vi "Configure Power Supply Rejection Ratio Analysis (Frequency).vi"(6 "Maximum Frequency (7: 20000000 Hz)":i32(ring)=7 items=["10", "100", "1000", "10000", "100000", "1000000", "10000000", "20000000"], 7 "Single Frequency (2: 100 Hz)":i32(ring)=2 items=["1", "10", "100", "1000", "10000", "100000", "1000000", "10000000", "2000000"], 8 "error in (no error)":errorcluster, 9 "Minimum Frequency (2: 100 Hz)":i32(ring)=2 items=["1", "10", "100", "1000", "10000", "100000", "1000000", "10000000", "2000000"], 10 "Frequency Mode (0: Sweep)":i32(ring) items=["Sweep", "Single"], 11 "VISA resource name":refnum<visa-resource-name>) -> (0 "error out":errorcluster, 3 "VISA resource name out":refnum<visa-resource-name>)   [LabVIEW 2015, in "Agilent 2000 3000 X-Series.lvlib"]
doc: "Configures the frequency for Power Supply Rejection Ratio (PSRR) power analysis.\n\n<b>Note:</b>\n - This VI is applicable for 3000T, 3000G, 4000, 6000 X-Series."
uses:
  Agilent 2000 3000 X-Series.lvlib
panel:
  # "Single Mode"
  # "Sweep Mode"
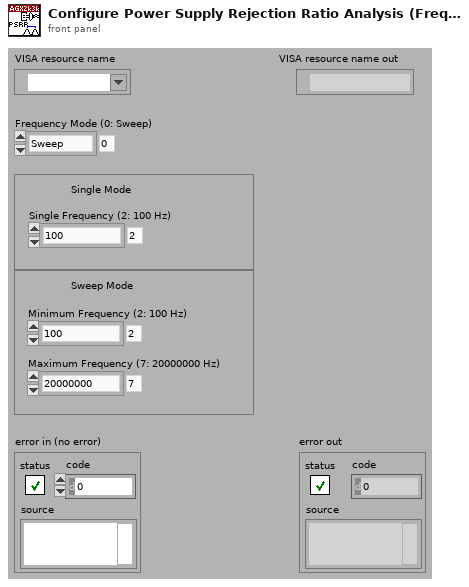
[diagram p1: front panel]
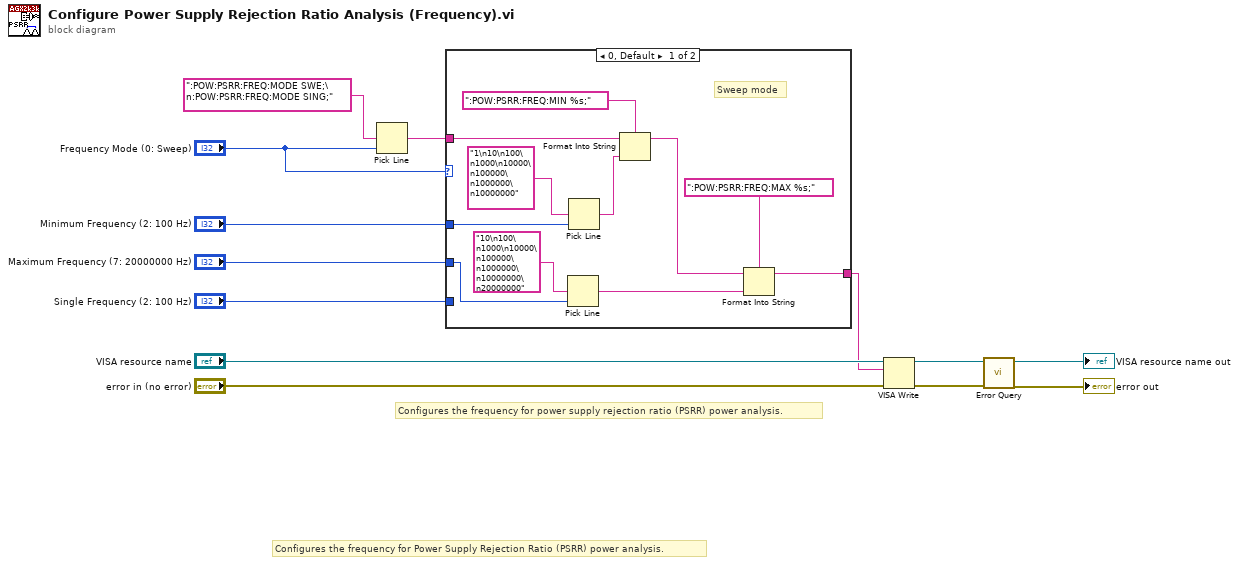
[diagram p0: block diagram]
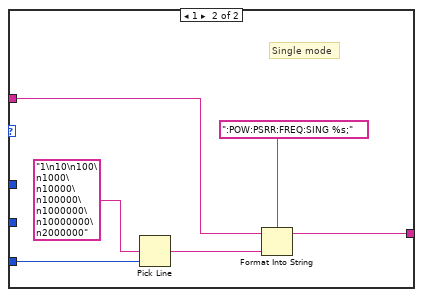
[diagram p2: hidden frame]
diagram:
  # "Configures the frequency for power supply rejection ratio (PSRR) power analysis."
  # "Configures the frequency for Power Supply Rejection Ratio (PSRR) power analysis."
  n1 = Pick Line(multi-line string=":POW:PSRR:FREQ:MODE SWE;\n:POW:PSRR:FREQ:MODE SING;", line index="Frequency Mode (0: Sweep)") -> (output string=w6:string)  [unwired: 1 in]
  n2 = case shown="0, Default" "Frequency Mode (0: Sweep)" {
    tunnel: w6 -> [w19 w29]
    tunnel: "Single Frequency (2: 100 Hz)" -> [_ w26]
    tunnel: [w20 w28] -> w1
    tunnel: "Minimum Frequency (2: 100 Hz)" -> [w18 _]
    tunnel: "Maximum Frequency (7: 20000000 Hz)" -> [w17 _]
    frame 0, Default {
      # "Sweep mode"
      n3 = Pick Line(multi-line string="10\n100\n1000\n10000\n100000\n1000000\n10000000\n20000000", line index=w17) -> (output string=w21:string)  [unwired: 1 in]
      n4 = Pick Line(multi-line string="1\n10\n100\n1000\n10000\n100000\n1000000\n10000000", line index=w18) -> (output string=w22:string)  [unwired: 1 in]
      n5 = Format Into String(format string=":POW:PSRR:FREQ:MIN %s;", initial string=w19, w22) -> (resulting string=w14:string)  [unwired: 1 in, 1 out]
      n6 = Format Into String(format string=":POW:PSRR:FREQ:MAX %s;", initial string=w14, w21) -> (resulting string=w20:string)  [unwired: 1 in, 1 out]
    }
    frame 1 {
      # "Single mode"
      n7 = Pick Line(multi-line string="1\n10\n100\n1000\n10000\n100000\n1000000\n10000000\n2000000", line index=w26) -> (output string=w25:string)  [unwired: 1 in]
      n8 = Format Into String(format string=":POW:PSRR:FREQ:SING %s;", initial string=w29, w25) -> (resulting string=w28:string)  [unwired: 1 in, 1 out]
    }
  }
  n9 = VISA Write(VISA resource name="VISA resource name", write buffer=w1, error in (no error)="error in (no error)") -> (VISA resource name out=w10:refnum<visa-resource-name>, error out=w9:errorcluster)  [unwired: 1 out]
  n10 = call "Error Query.vi"("error in (no error)"=w9, "VISA resource name"=w10) -> ("error out"=→"error out":errorcluster, "VISA resource name out"=→"VISA resource name out":refnum<visa-resource-name>)  [unwired: 6 in, 2 out]
